vi "Day1Part2.vi"() -> ()   [LabVIEW 2024]
uses:
  <vilib>/Utility/file.llb/Read Delimited Spreadsheet (I64).vi
panel:
  out "sum":i64
  out "all rows":i64[][](array[numeric])
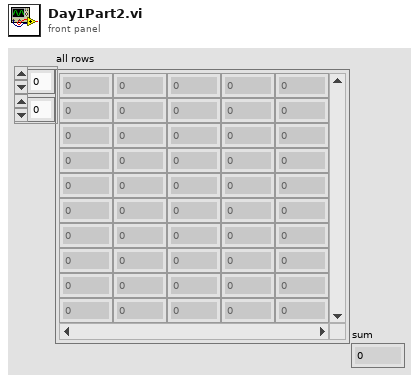
[diagram p1: front panel]
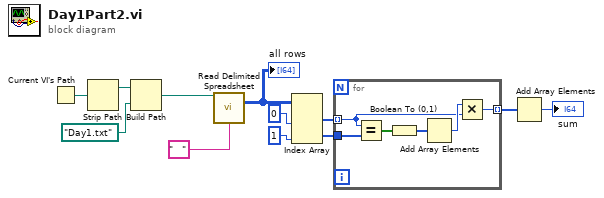
[diagram p0: block diagram]
diagram:
  n1 = Current VI's Path() -> (path=w12:path)
  n2 = Strip Path(path=w12) -> (stripped path=w11:path)  [unwired: 1 out]
  n3 = Build Path(base path=w11, name or relative path=path "Day1.txt") -> (appended path=w9:path)
  n4 = call-poly <vilib>:"Read Delimited Spreadsheet.vi"("file path (dialog if empty)"=w9, "delimiter (\\t)"="   " ("delimiter (\\t)")) -> ("all rows"=w6:i64[][])  [unwired: 8 in, 5 out]
  "all rows" <- w6
  n5 = Index Array(array=w6, index (col) #1=0 ("disabled index (col)"), index (col) #2=1 ("index (col)")) -> (element #1=w3:i64[], element #2=w2:i64[])  [unwired: 2 in]
  n6 = for {
    tunnel: w3 -> [w14] mode=indexing
    tunnel: w2 -> [w18]
    tunnel: [w13] -> w1 mode=indexing
    n7 = Equal?(x=w14, y=w18) -> (x = y?=w17:bool[])
    n8 = Boolean To (0,1)(Boolean=w17) -> (0, 1=w16:i16[])
    n9 = Add Array Elements(numeric array=w16) -> (sum=w15:i16)
    n10 = Multiply(x=w15, y=w14) -> (x*y=w13:i64)
  }
  n11 = Add Array Elements(numeric array=w1) -> (sum=→"sum":i64)
